vi "Read Current Step.vi"(8 "error in (no error)":errorcluster, 11 "Scanner.lvclass in":refnum<class "Scanner.lvclass">) -> (0 "error out":errorcluster, 1 "Ind Vars[i]":dbl, 2 "Current Step":u32, 3 "Scanner.lvclass out":refnum<class "Scanner.lvclass">)   [LabVIEW 2012, in "Scanner.lvclass"]
doc: "(Dynamic) Return the current position (actual, not intended) of this Scanner."
uses:
  Scanner.lvclass
  Scanner.lvclass/Scanner.ctl
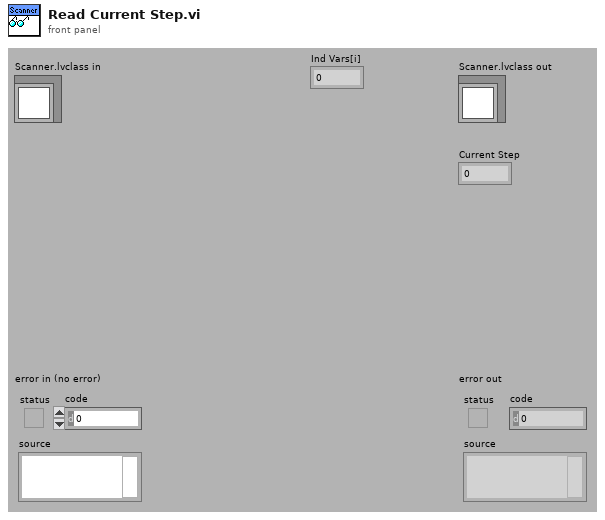
[diagram p1: front panel]
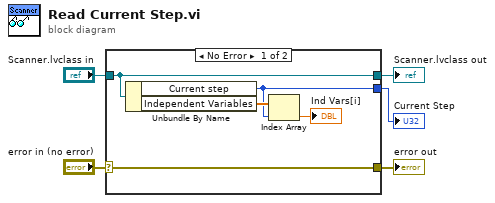
[diagram p0: block diagram]
diagram:
  n1 = case shown="No Error" "error in (no error)" {
    selector: "error in (no error)" -> [w10 w11]
    tunnel: [w10 w11] -> w4
    tunnel: [w9 w12] -> w2
    tunnel: "Scanner.lvclass in" -> [w9 w12]
    tunnel: [w7 _] -> w1
    frame No Error {
      n2 = Unbundle By Name(w9) -> ("Current step"=w7:u32, "Independent Variables"=w8:dbl[])
      n3 = Index Array(array=w8, index=w7) -> (element=→"Ind Vars[i]":dbl)
    }
    frame Error {
    }
  }
  "error out" <- w4
  "Scanner.lvclass out" <- w2
  "Current Step" <- w1
